vi "Function_Block Spot #2.vi"(6 "Center(Annulus)":cluster{"X":sgl, "Y":sgl} {"Y" format="%.2f"; "X" format="%.2f"}, 8 "Error in":errorcluster, 9 "CoordSys In":T2 {"Measurement System"."Axis Reference" items=["Direct", "Indirect"]; "Measurement System"."Angle (deg)" format="%.2f"; "Measurement System"."Origin"."Y" format="%.2f"; "Measurement System"."Origin"."X" format="%.2f"; "Reference System"."Axis Reference" items=["Direct", "Indirect"]; "Reference System"."Angle (deg)" format="%.2f"; "Reference System"."Origin"."Y" format="%.2f"; "Reference System"."Origin"."X" format="%.2f"}, 10 "Data Cluster In":cluster{"Name":string, "Variant In":variant}, 11 "Image Dst In":T4) -> (0 "Error out":errorcluster, 2 "ROI out":T1 {"Contours"."Type" items=["No Selection", "Point", "Line", "Rectangle", "Oval", "Polygon", "Freehand Region", "Annulus", "Unused2", "Unused3", "Broken Line", "Freehand Line", "Rotated Rectangle"]}, 3 "Objects":T3(array[cluster]) {"Area" format="%.2f"; "Object Center"."Y" format="%.2f"; "Object Center"."X" format="%.2f"})   [LabVIEW 2013]
uses:
  <vilib>/vision/Image Controls.llb/IMAQ Image.ctl
  Control/Control_Block Spot.ctl
  <vilib>/vision/NI_Vision_Development_Module.lvlib
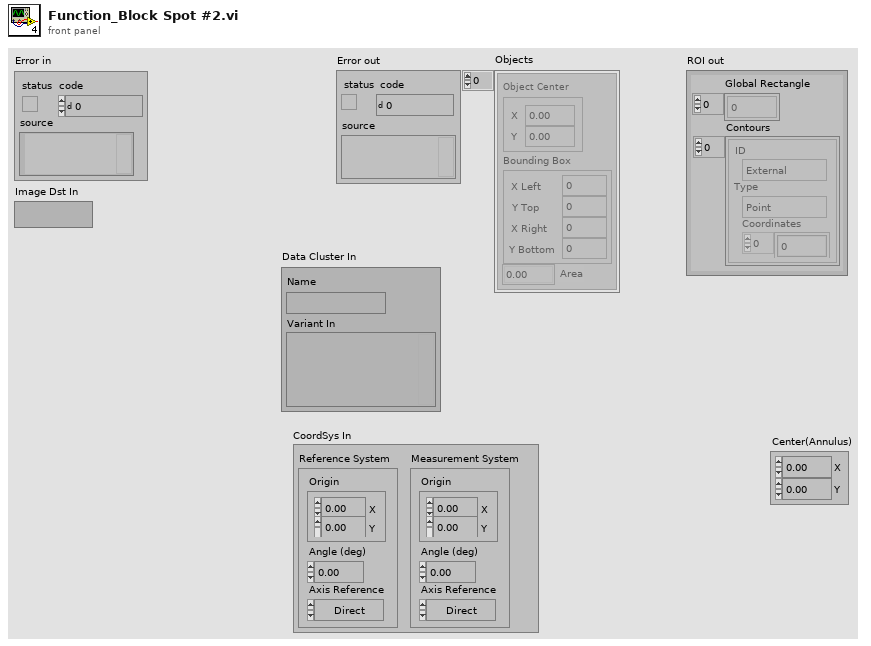
[diagram p1: front panel]
types:
  T1 = typedef "ROI Descriptor" = cluster{"Global Rectangle":i32[], "Contours":cluster{"ID":enum32{"External", "Internal"}, "Type":u32, "Coordinates":i32[]}[]}
  T2 = typedef "IMAQ Coordinate System" = cluster{"Reference System":cluster{"Origin":cluster{"X":sgl, "Y":sgl}, "Angle (deg)":sgl, "Axis Reference":u32}, "Measurement System":cluster{"Origin":cluster{"X":sgl, "Y":sgl}, "Angle (deg)":sgl, "Axis Reference":u32}}
  T3 = cluster{"Object Center":cluster{"X":dbl, "Y":dbl}, "Bounding Box":cluster{"X Left":dbl, "Y Top":dbl, "X Right":dbl, "Y Bottom":dbl}, "Area":dbl}[]
  T4 = typedef "IMAQ Image.ctl" = refnum<image>
  T5 = typedef "Control_Block Spot.ctl" = cluster{"Name":string, "ROI":cluster{"Global Rectangle":i32[], "Contours":cluster{"ID":enum32{"External", "Internal"}, "Type":u32, "Coordinates":i32[]}[]}, "Magnification(黑點)":i32, "Settings(黑點)":cluster{"Objects":enum16{"Bright Objects", "Dark Objects"}, "Threshold":i32, "Min Object Size":bool, "Min Size":i32, "Max Object Size":bool, "Max Size":i32}, "Highlight":cluster{"Kernel Size":i32, "Divider":sgl, "Min Object Size":bool}}
  T6 = cluster{"Global Rectangle":i32[], "Contours":cluster{"ID":enum32{"External", "Internal"}, "Type":u32, "Coordinates":i32[]}[]}
  T7 = cluster{"Objects":enum16{"Bright Objects", "Dark Objects"}, "Threshold":i32, "Min Object Size":bool, "Min Size":i32, "Max Object Size":bool, "Max Size":i32}
  T8 = cluster{"ID":enum32{"External", "Internal"}, "Type":u32, "Coordinates":i32[]}[]
  T9 = cluster{"ID":enum32{"External", "Internal"}, "Type":u32, "Coordinates":i32[]}
  T10 = cluster{"Origin":cluster{"X":sgl, "Y":sgl}, "Angle (deg)":sgl, "Axis Reference":u32}
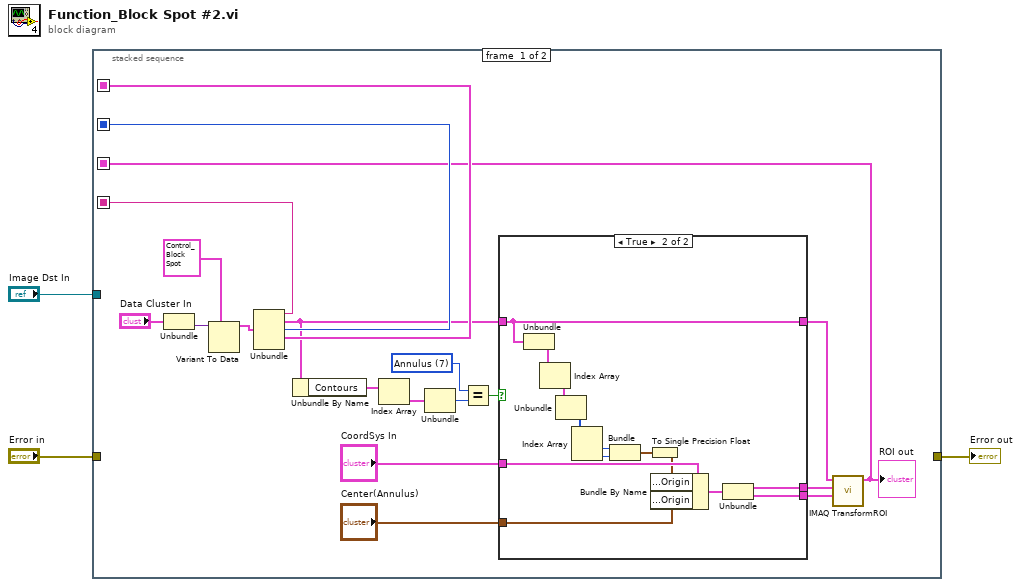
[diagram p0: block diagram]
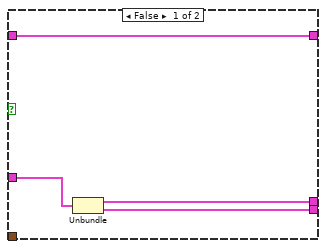
[diagram p2: hidden frame]
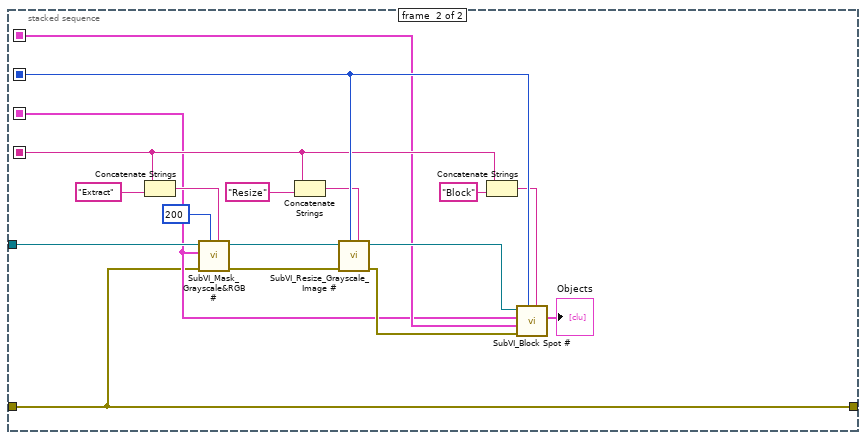
[diagram p3: hidden frame]
diagram:
  n1 = stacked-sequence {
    seq-local: [w18 _] -> [_ w47]
    seq-local: [w5 _] -> [_ w43]
    seq-local: [w17 _] -> [_ w54]
    seq-local: [w16 _] -> [_ w45]
    tunnel: [_ w42] -> w3
    tunnel: "Error in" -> [_ w42]
    tunnel: "Image Dst In" -> [_ w46]
    frame #0 {
      w12 = u32 7 items=["No Selection", "Point", "Line", "Rectangle", "Oval", "Polygon", "Freehand Region", "Annulus", "Unused2", "Unused3", "Broken Line", "Freehand Line", "Rotated Rectangle"] ("Type")
      n2 = Unbundle("Data Cluster In") -> ("Variant In"=w21:variant)  [unwired: 1 out]
      n3 = Variant To Data(type=T5 {"Name"="", "ROI"={"Global Rectangle"=[], "Contours"=[]}, "Magnification(黑點)"=0, "Settings(黑點)"={"Objects"=enum."Bright Objects", "Threshold"=0, "Min Object Size"=FALSE, "Min Size"=0, "Max Object Size"=FALSE, "Max Size"=0}, "Highlight"={"Kernel Size"=0, "Divider"=0.0, "Min Object Size"=FALSE}} ("黑點_Setting"), Variant=w21) -> (data=w22:T5)  [unwired: 1 in, 1 out]
      n4 = Unbundle(w22) -> ("Name"=w18:string, "ROI"=w9:T6, "Magnification(黑點)"=w17:i32, "Settings(黑點)"=w16:T7)  [unwired: 1 out]
      n5 = Unbundle By Name(w9) -> ("Contours"=w14:T8)
      n6 = Index Array(array=w14) -> (element=w13:T9)  [unwired: 1 in]
      n7 = Unbundle(w13) -> ("Type"=w11:u32)  [unwired: 2 out]
      n8 = Equal?(x=w12, y=w11) -> (x = y?=w10:bool)
      n9 = case shown="True" w10 {
        tunnel: "CoordSys In" -> [w26 w36]
        tunnel: [w23 w35] -> w8
        tunnel: w9 -> [w23 w35]
        tunnel: [w25 w28] -> w7
        tunnel: [w24 w27] -> w6
        tunnel: "Center(Annulus)" -> [_ w32]
        frame False {
          n10 = Unbundle(w26) -> ("Reference System"=w25:T10, "Measurement System"=w24:T10)
        }
        frame True {
          n11 = Unbundle(w35) -> ("Contours"=w39:T8)  [unwired: 1 out]
          n12 = Index Array(array=w39) -> (element=w37:T9)  [unwired: 1 in]
          n13 = Unbundle(w37) -> ("Coordinates"=w38:i32[])  [unwired: 2 out]
          n14 = Index Array(array=w38) -> (element #1=w34:i32, element #2=w33:i32)  [unwired: 2 in]
          n15 = Bundle(w34, w33) -> (w31:cluster{i32, i32})  [unwired: 1 in]
          n16 = To Single Precision Float(number=w31) -> (single precision float=w30:cluster{sgl, sgl})
          n17 = Bundle By Name(cluster=w36, "Reference System.Origin"=w30, "Measurement System.Origin"=w32) -> (w29:T2)
          n18 = Unbundle(w29) -> ("Reference System"=w28:T10, "Measurement System"=w27:T10)
        }
      }
      n19 = call "IMAQ TransformROI"("New Reference"=w6, "Base Reference"=w7, "ROI Descriptor"=w8) -> ("ROI Descriptor out"=w5:T1)  [unwired: 7 in, 1 out]
      "ROI out" <- w5
    }
    frame #1 {
      n20 = Concatenate Strings(w47, "Extract" ("Image Register Name")) -> (w52:string)
      n21 = call "SubVI_Mask_Grayscale&RGB #.vi"("Image Register Name"=w52, "Background Value"=200, "Error in"=w42, "ROI Descriptor"=w43, "Image Src In"=w46) -> ("Error out"=w57:errorcluster, "Image Dst Out"=w56:T4)  [unwired: 4 in, 1 out]
      n22 = Concatenate Strings(w47, "Resize" ("Image Register Name")) -> (w50:string)
      n23 = call "SubVI_Resize_Grayscale_Image #.vi"("Image Register Name"=w50, "Magnification"=w54, "Error In"=w57, "Image In"=w56) -> ("Error Out"=w44:errorcluster, "Image Out"=w55:T4)  [unwired: 5 in, 1 out]
      n24 = Concatenate Strings(w47, "Block" ("string")) -> (w49:string)
      n25 = call "SubVI_Block Spot #.vi"("Image Register Name"=w49, "Magnification"=w54, "Error in"=w44, "Settings"=w45, "ROI Descriptor"=w43, "Image In"=w55) -> ("Objects"=→"Objects":T3)  [unwired: 4 in, 1 out]
    }
  }
  "Error out" <- w3
